vi "Modificar_Arreglos(SubVi).vi"(1 "Selector de Variable":T5, 2 "input cluster":T1={"Opción X"=0, "Opción Y"=0, "Opción Z"=0, "Posición X"=0.0, "Velocidad X"=0.0, "Posición Y"=0.0, "Velocidad Y"=0.0, "Posición Z"=0.0, "Velocidad Z"=0.0, "Escala"=[[1.0, 1.0, 1.0], [1.0, 1.0, 1.0], [1.0, 1.0, 1.0]], "Translación"=[[1.0, 1.0, 0.0], [0.0, 0.0, 0.0], [0.0, 0.0, 0.0]], "Rotación"=[[1.0, 0.0, 0.0, 0.0], [1.0, 0.0, 0.0, 0.0], [1.0, 0.0, 0.0, 0.0]], "Operacion SX"=enum."Escala", "Eje de la Figura SX"=enum."X", "Figura Geométrica SX"=enum."Cono", "Operacion SY"=enum."Escala", "Eje de la Figura SY"=enum."X", "Figura Geométrica SY"=enum."Cono", "Operacion SZ"=enum."Escala", "Eje de la Figura SZ"=enum."X", "Figura Geométrica SZ"=enum."Cono"}) -> (0 "output cluster":T1={"Opción X"=0, "Opción Y"=0, "Opción Z"=0, "Posición X"=0.0, "Velocidad X"=0.0, "Posición Y"=0.0, "Velocidad Y"=0.0, "Posición Z"=0.0, "Velocidad Z"=0.0, "Escala"=[[1.0, 1.0, 1.0], [1.0, 1.0, 1.0], [1.0, 1.0, 1.0]], "Translación"=[[1.0, 1.0, 0.0], [0.0, 0.0, 0.0], [0.0, 0.0, 0.0]], "Rotación"=[[1.0, 0.0, 0.0, 0.0], [1.0, 0.0, 0.0, 0.0], [1.0, 0.0, 0.0, 0.0]], "Operacion SX"=enum."Escala", "Eje de la Figura SX"=enum."X", "Figura Geométrica SX"=enum."Cono", "Operacion SY"=enum."Escala", "Eje de la Figura SY"=enum."X", "Figura Geométrica SY"=enum."Cono", "Operacion SZ"=enum."Escala", "Eje de la Figura SZ"=enum."X", "Figura Geométrica SZ"=enum."Cono"})   [LabVIEW 2017]
uses:
  Control_Opciones.ctl
  Control_Operacion.ctl
  Control_Eje_Figura.ctl
  Control_Figura.ctl
  Control_Selector_Variable.ctl
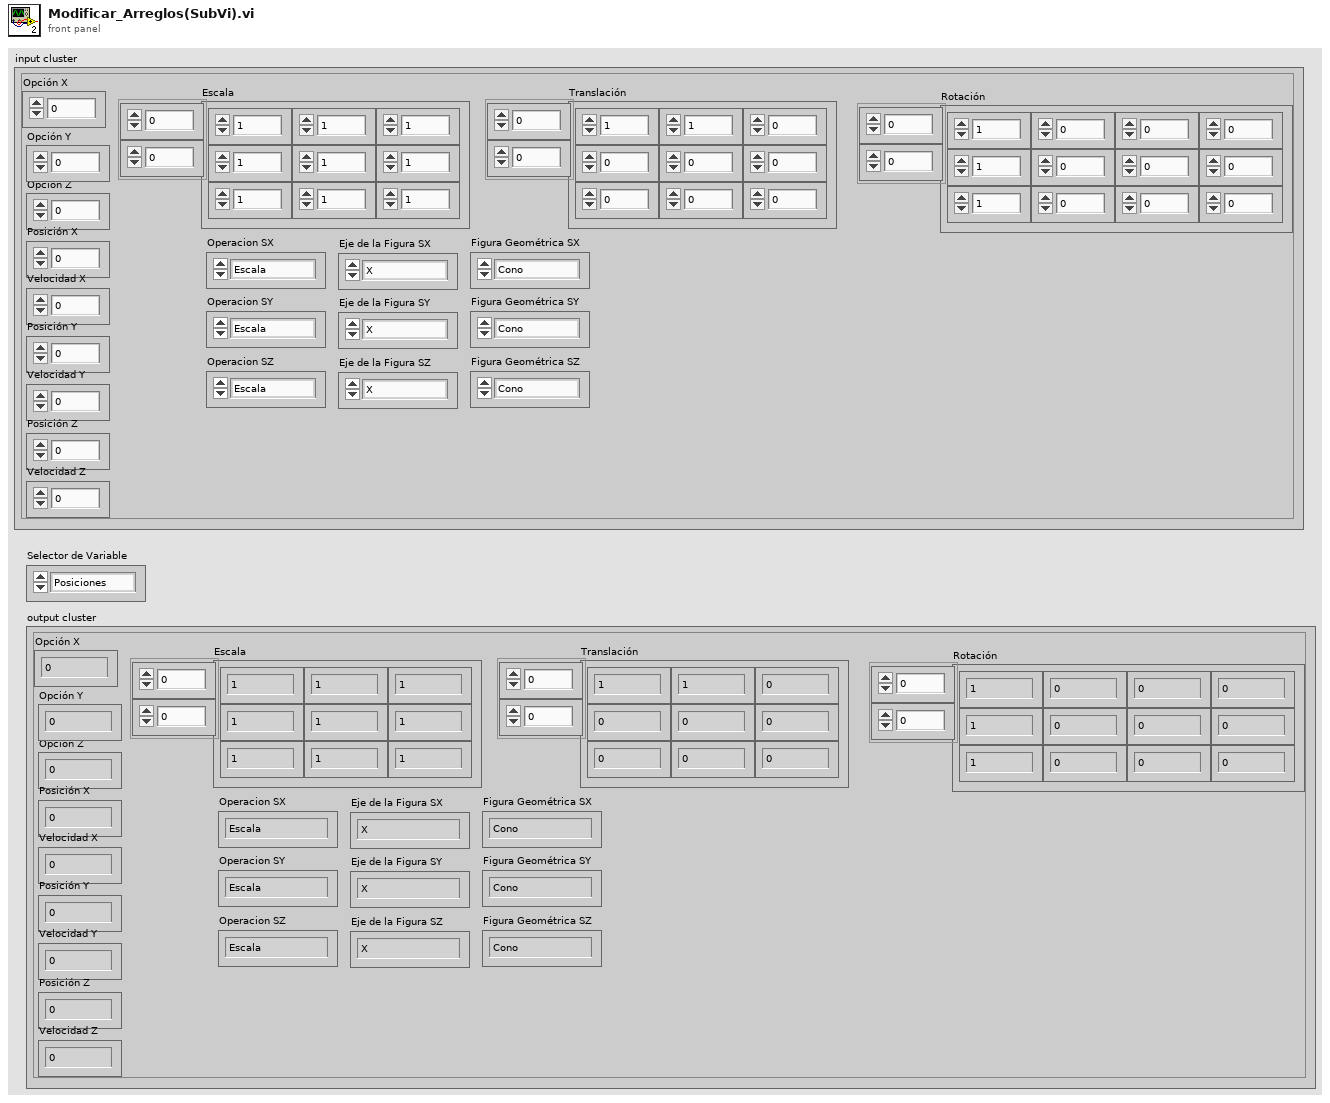
[diagram p1: front panel]
types:
  T1 = typedef "Control_Opciones.ctl" = cluster{"Opción X":i32, "Opción Y":i32, "Opción Z":i32, "Posición X":dbl, "Velocidad X":dbl, "Posición Y":dbl, "Velocidad Y":dbl, "Posición Z":dbl, "Velocidad Z":dbl, "Escala":dbl[][], "Translación":dbl[][], "Rotación":dbl[][], "Operacion SX":T2, "Eje de la Figura SX":T3, "Figura Geométrica SX":T4, "Operacion SY":T2, "Eje de la Figura SY":T3, "Figura Geométrica SY":T4, "Operacion SZ":T2, "Eje de la Figura SZ":T3, "Figura Geométrica SZ":T4}
  T2 = typedef "Control_Operacion.ctl" = enum16{"Escala", "Translación", "Rotación"}
  T3 = typedef "Control_Eje_Figura.ctl" = enum16{"X", "Y", "Z"}
  T4 = typedef "Control_Figura.ctl" = enum16{"Cono", "Esfera", "Cilindro"}
  T5 = typedef "Control_Selector_Variable.ctl" = enum16{"Posiciones", "Velocidades"}
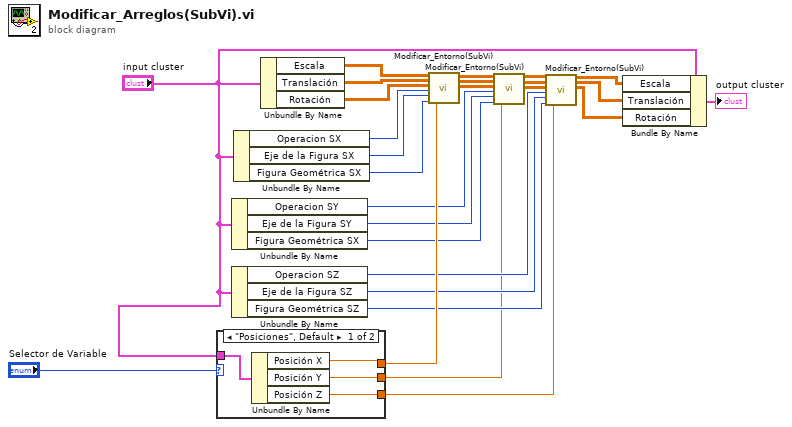
[diagram p0: block diagram]
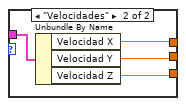
[diagram p2: hidden frame]
diagram:
  n1 = case shown="\"Posiciones\", Default" "Selector de Variable" {
    tunnel: "input cluster" -> [w31 w35]
    tunnel: [w30 w34] -> w20
    tunnel: [w29 w33] -> w7
    tunnel: [w28 w32] -> w6
    frame "Posiciones", Default {
      n2 = Unbundle By Name(w31) -> ("Posición X"=w30:dbl, "Posición Y"=w29:dbl, "Posición Z"=w28:dbl)
    }
    frame "Velocidades" {
      n3 = Unbundle By Name(w35) -> ("Velocidad X"=w34:dbl, "Velocidad Y"=w33:dbl, "Velocidad Z"=w32:dbl)
    }
  }
  n4 = Unbundle By Name("input cluster") -> ("Operacion SY"=w16:T2, "Eje de la Figura SY"=w15:T3, "Figura Geométrica SX"=w14:T4)
  n5 = Unbundle By Name("input cluster") -> ("Operacion SZ"=w10:T2, "Eje de la Figura SZ"=w9:T3, "Figura Geométrica SZ"=w8:T4)
  n6 = Unbundle By Name("input cluster") -> ("Operacion SX"=w24:T2, "Eje de la Figura SX"=w23:T3, "Figura Geométrica SX"=w22:T4)
  n7 = Unbundle By Name("input cluster") -> ("Escala"=w27:dbl[][], "Translación"=w26:dbl[][], "Rotación"=w25:dbl[][])
  n8 = call "Modificar_Entorno(SubVi).vi"("Escala"=w27, "Translación"=w26, "Rotación"=w25, "Operación"=w24, "Eje de la Figura"=w23, "Figura Geometrica"=w22, "Valor"=w20) -> ("Escala Salida"=w19:dbl[][], "Translación Salida"=w18:dbl[][], "Rotación Salida"=w17:dbl[][])  [unwired: 10 in]
  n9 = call "Modificar_Entorno(SubVi).vi"("Escala"=w19, "Translación"=w18, "Rotación"=w17, "Operación"=w16, "Eje de la Figura"=w15, "Figura Geometrica"=w14, "Valor"=w7) -> ("Escala Salida"=w13:dbl[][], "Translación Salida"=w12:dbl[][], "Rotación Salida"=w11:dbl[][])  [unwired: 10 in]
  n10 = call "Modificar_Entorno(SubVi).vi"("Escala"=w13, "Translación"=w12, "Rotación"=w11, "Operación"=w10, "Eje de la Figura"=w9, "Figura Geometrica"=w8, "Valor"=w6) -> ("Escala Salida"=w4:dbl[][], "Translación Salida"=w3:dbl[][], "Rotación Salida"=w2:dbl[][])  [unwired: 10 in]
  n11 = Bundle By Name(cluster="input cluster", "Escala"=w4, "Translación"=w3, "Rotación"=w2) -> (→"output cluster":T1)
